vi "fft -- tdo thing -- V1.vi"(0 "power spectra":cluster{"f0":dbl, "df":dbl, "magnitude":dbl[]}[](array[cluster]) {"magnitude" format="%.2p"; "f0" format="%.2p"; "df" format="%.2p"}, 1 "fft -- action":T2, 3 "tdms file":refnum<k34>, 5 "Data window IN":T1={"Start"=39994, "Length"=13169, "Channel numbers"=[0], "Channel names"=["freq", ""], "Group name"="p"}, 11 "time (sec)":dbl=0.07527795000000001 format="%#_3p", 12 "range min":dbl=0.07527795000000001 format="%#_3p", 14 "range max":dbl=0.07527795000000001 format="%#_3p") -> (4 "amp":dbl=0.011117700000000001 format="%#_3p", 6 "freq":dbl=0.011117700000000001 format="%#_8p", 15 "XY Graph":cluster{dbl[], dbl[]}(graph))   [LabVIEW 2021]
uses:
  fft -- tdo thing -- control.vi.ctl
  fft -- data win.ctl
  Read TDMS waveform -- control.vi.ctl
  <vilib>/Analysis/4window.llb/Hanning Window (DBL).vi
  <vilib>/Analysis/2dsp.llb/1D Convolution (DBL).vi
  <vilib>/Analysis/4window.llb/AllCosWindow (DBL).vi
  <vilib>/Analysis/NI_AALPro.lvlib
  <vilib>/Analysis/NI_AAL_SigProc.lvlib
panel:
  # "OR"
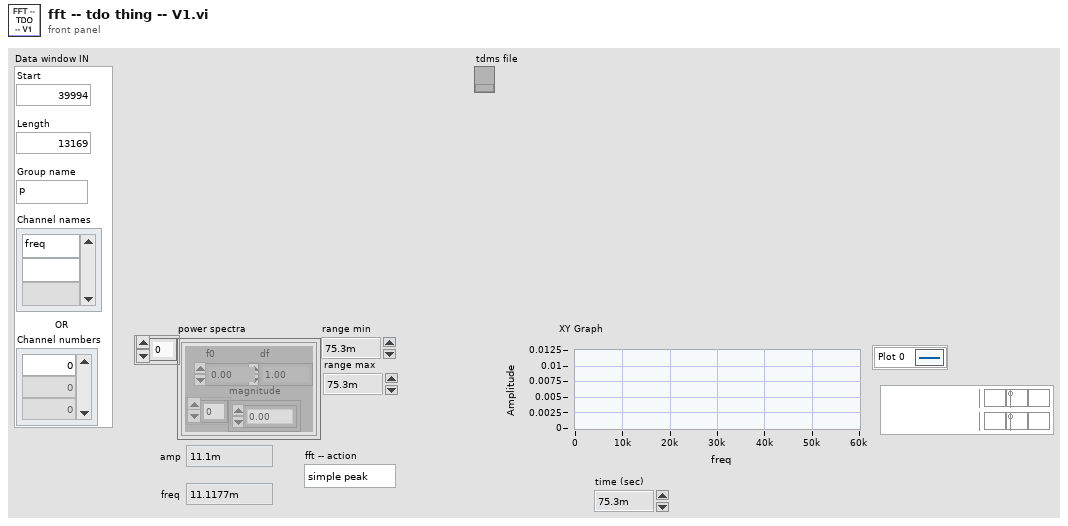
[diagram p1: front panel]
types:
  T1 = typedef "fft -- data win.ctl" = cluster{"Start":i64, "Length":i32, "Channel numbers":i64[], "Channel names":string[], "Group name":string}
  T2 = typedef "fft -- tdo thing -- control.vi.ctl" = enum16{"simple peak", "to array", "tdo thing", "tdo -- convo"}
  T3 = typedef "Read TDMS waveform -- control.vi.ctl" = enum16{"read", "open", "close"}
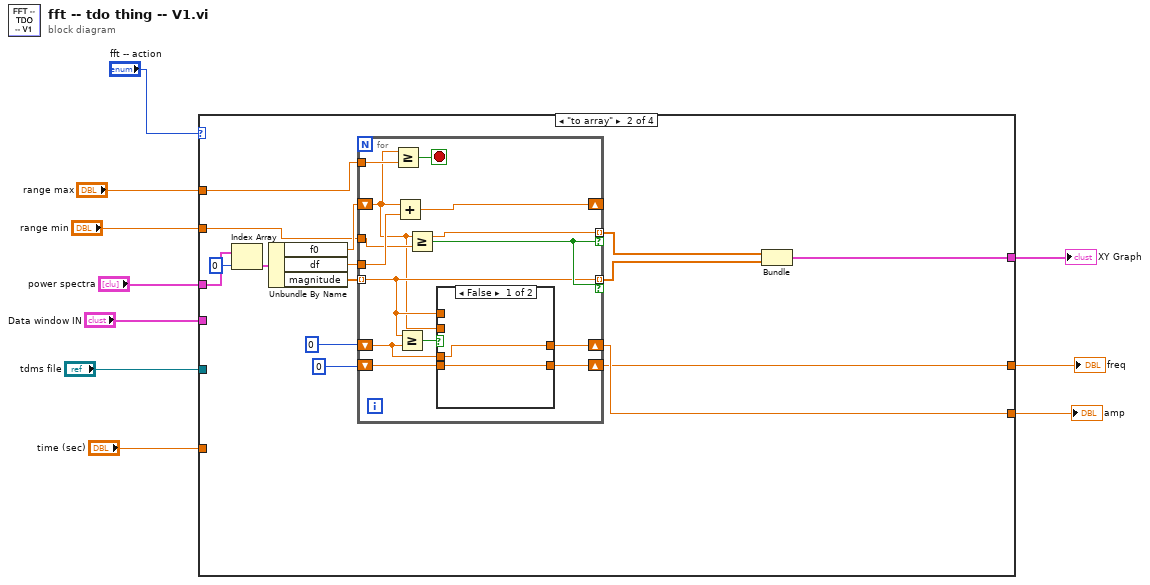
[diagram p0: block diagram]
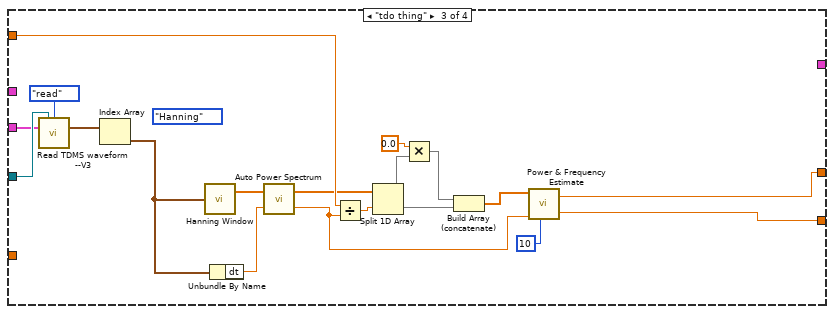
[diagram p4: hidden frame]
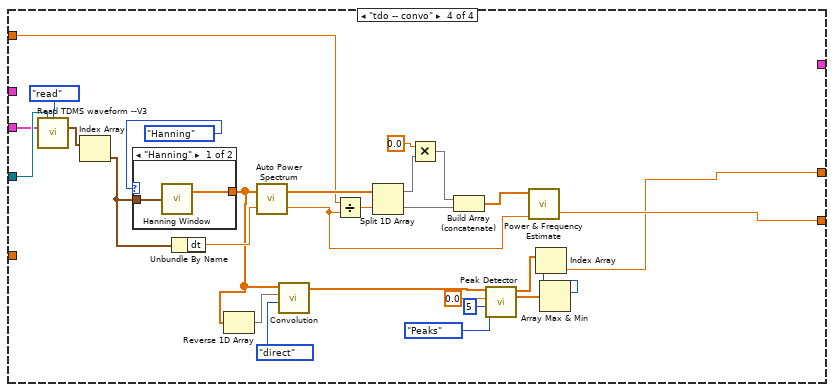
[diagram p5: hidden frame]
diagram:
  n1 = case shown="\"to array\"" "fft -- action" {
    tunnel: "power spectra" -> [_ w25 _ _]
    tunnel: "time (sec)" -> [_ _ _ _]
    tunnel: "range max" -> [_ w17 _ _]
    tunnel: "range min" -> [_ w16 w56 w71]
    tunnel: [_ w13 w55 w84] -> w8
    tunnel: [_ w11 w44 w62] -> w1
    tunnel: [_ w12 _ _] -> w4
    tunnel: "tdms file" -> [_ _ w60 w88]
    tunnel: "Data window IN" -> [_ _ w59 w87]
    frame "simple peak", Default {
    }
    frame "to array" {
      n2 = Index Array(array=w25, index=0) -> (element=w23:cluster{"f0":dbl, "df":dbl, "magnitude":dbl[]})
      n3 = Unbundle By Name(w23) -> ("f0"=w21:dbl, "df"=w20:dbl, "magnitude"=w22:dbl[])
      n4 = for {
        tunnel: w22 -> [w29] mode=indexing
        tunnel: [w29] -> w18 mode=indexing if=w35
        shift-right: [w38] -> _
        shift-left: w21 -> [w27]
        tunnel: [w27] -> w19 mode=indexing if=w35
        tunnel: w20 -> [w37]
        tunnel: w17 -> [w34]
        tunnel: w16 -> [w33]
        shift-right: [w30] -> w13
        shift-left: i64 0 ("Start") -> [w31]
        shift-right: [w28] -> w11
        shift-left: i64 0 ("Start") -> [w26]
        stop <- w36 stop-if-true
        n5 = Greater Or Equal?(x=w27, y=w34) -> (x >= y?=w36:bool)
        n6 = Add(x=w27, y=w37) -> (x+y=w38:dbl)
        n7 = Greater Or Equal?(x=w29, y=w31) -> (x >= y?=w32:bool)
        n8 = Greater Or Equal?(x=w27, y=w33) -> (x >= y?=w35:bool)
        n9 = case shown="False" w32 {
          tunnel: w31 -> [w40 _]
          tunnel: [w40 w42] -> w30
          tunnel: w29 -> [_ w42]
          tunnel: [w39 w41] -> w28
          tunnel: w27 -> [_ w41]
          tunnel: w26 -> [w39 _]
          frame False {
          }
          frame True {
          }
        }
      }
      n10 = Bundle(w19, w18) -> (w12:cluster{dbl[], dbl[]})  [unwired: 1 in]
    }
    frame "tdo thing" {
      (unwired) enum16{"Hanning", "Box", "Blackman"}."Hanning" ("window type")
      n11 = call "Read TDMS waveform --V3.vi"("tdms file in"=w60, "TDMS"=Read_TDMS_waveform_--_control.vi."read", "Data window IN"=w59) -> ("Data out"=w58:waveform(dbl)[])  [unwired: 7 in, 5 out]
      n12 = Index Array(array=w58) -> (element=w57:waveform(dbl))  [unwired: 1 in]
      n13 = call-poly <vilib>:"Hanning Window.vi"("X"=w57) -> ("Windowed X"=w54:dbl[])  [unwired: 1 out]
      n14 = Unbundle By Name(w57) -> ("dt"=w53:dbl)
      n15 = call <vilib>:"Auto Power Spectrum.vi"("dt"=w53, "Signal (V)"=w54) -> ("df"=w46:dbl, "Power Spectrum (V^2 rms)"=w52:dbl[])
      n16 = Divide(x=w56, y=w46) -> (x/y=w51:dbl)
      n17 = Split 1D Array(array=w52, index=w51) -> (first subarray=w48:dbl[], second subarray=w50:dbl[])
      n18 = Multiply(x=0.0 ("element"), y=w48) -> (x*y=w47:dbl[])
      n19 = Build Array (concatenate)(w47, w50) -> (w45:dbl[])
      n20 = call <vilib>:"Power & Frequency Estimate.vi"("span"=10, "df"=w46, "Power Spectrum (V^2 rms)"=w45) -> ("est power peak"=w55:dbl, "est frequency peak"=w44:dbl)  [unwired: 2 in, 1 out]
    }
    frame "tdo -- convo" {
      n21 = call "Read TDMS waveform --V3.vi"("tdms file in"=w88, "TDMS"=Read_TDMS_waveform_--_control.vi."read", "Data window IN"=w87) -> ("Data out"=w86:waveform(dbl)[])  [unwired: 7 in, 5 out]
      n22 = Index Array(array=w86) -> (element=w85:waveform(dbl))  [unwired: 1 in]
      n23 = case shown="\"Hanning\"" enum16{"Hanning", "Box", "Blackman"}."Hanning" ("window type") {
        tunnel: [w91 w92] -> w74
        tunnel: w85 -> [w90 w92]
        frame "Hanning" {
          n24 = call-poly <vilib>:"Hanning Window.vi"("X"=w90) -> ("Windowed X"=w91:dbl[])  [unwired: 1 out]
        }
        frame "Box", Default {
        }
      }
      n25 = Unbundle By Name(w85) -> ("dt"=w83:dbl)
      n26 = Reverse 1D Array(array=w74) -> (reversed array=w73:dbl[])
      n27 = call <vilib>:"Auto Power Spectrum.vi"("dt"=w83, "Signal (V)"=w74) -> ("df"=w70:dbl, "Power Spectrum (V^2 rms)"=w82:dbl[])
      n28 = call-poly <vilib>:"Convolution.vi"("algorithm"=enum32{"direct", "frequency domain"}."direct", "Y"=w73, "X"=w74) -> ("X * Y"=w69:dbl[])  [unwired: 7 in, 1 out]
      n29 = Divide(x=w71, y=w70) -> (x/y=w81:dbl)
      n30 = Split 1D Array(array=w82, index=w81) -> (first subarray=w78:dbl[], second subarray=w80:dbl[])
      n31 = Multiply(x=0.0 ("element"), y=w78) -> (x*y=w77:dbl[])
      n32 = Build Array (concatenate)(w77, w80) -> (w76:dbl[])
      n33 = call <vilib>:"Peak Detector.vi"("peaks/valleys"=enum32{"Peaks", "Valleys"}."Peaks", "width"=5, "threshold"=0.0, "X"=w69) -> ("Amplitudes"=w65:dbl[], "Locations"=w63:dbl[])  [unwired: 3 in, 3 out]
      n34 = call <vilib>:"Power & Frequency Estimate.vi"("df"=w70, "Power Spectrum (V^2 rms)"=w76) -> ("est power peak"=w84:dbl)  [unwired: 3 in, 2 out]
      n35 = Array Max & Min(array=w65) -> (max index (indices)=w64:i32)  [unwired: 3 out]
      n36 = Index Array(array=w63, index=w64) -> (element=w62:dbl)
    }
  }
  "XY Graph" <- w4
  "amp" <- w8
  "freq" <- w1
